vi "Analog Input - 1 Channel - N Samples.vi"() -> ()   [LabVIEW 2019]
uses:
  <vilib>/myRIO/Common/Instrument Driver Framework/ELVIS III v1.0/AI Block/vis/ELVIS III v1.0 AI Block Read.vi
  <vilib>/myRIO/Common/Instrument Driver Framework/ELVIS III v1.0/AI Block/vis/ELVIS III v1.0 Close AI Block.vi
  <vilib>/myRIO/Common/Instrument Driver Framework/myRIO v1.0/UART/vis/myRIO v1.0 Close UART.vi
  <vilib>/myRIO/Common/Instrument Driver Framework/Utilities/vis/Sample Rate To Ticks.vi
  <vilib>/myRIO/Common/Instrument Driver Framework/ELVIS III v1.0/AI Block/vis/ELVIS III v1.0 Unreserve AI Block.vi
  <vilib>/myRIO/Common/Instrument Driver Framework/ELVIS III v1.0/AI Block/vis/ELVIS III v1.0 Build MUX Configuration AI Block.vi
  <vilib>/Utility/error.llb/Error Cluster From Error Code.vi
  <vilib>/myRIO/Common/Instrument Driver Framework/myRIO v1.0/Resource Manager/vis/myRIO v1.0 Block Write Configuration.vi
  <vilib>/myRIO/Common/Instrument Driver Framework/ELVIS III v1.0/AI Block/vis/ELVIS III v1.0 AI Block Read Bank A.vi
  <vilib>/myRIO/Common/Instrument Driver Framework/ELVIS III v1.0/AI Block/vis/ELVIS III v1.0 AI Block Read Bank B.vi
  <vilib>/myRIO/Common/Instrument Driver Framework/ELVIS III v1.0/Resource Manager/vis/ELVIS III v1.0 Unreserve Channel List.vi
  <vilib>/myRIO/Common/Instrument Driver Framework/myRIO v1.0/myRIO v1.0 Close.vi
  <vilib>/myRIO/Common/Instrument Driver Framework/Utilities/vis/FPGA Ref Manager.vi
  <vilib>/myRIO/Common/Instrument Driver Framework/ELVIS III v1.0/ELVIS III v1.0 Reset FPGA.vi
  <vilib>/myRIO/Common/Instrument Driver Framework/myRIO v1.0/IRQ/vis/myRIO v1.0 IRQ Info FGV.vi
  <vilib>/myRIO/Common/Instrument Driver Framework/myRIO v1.0/IRQ/vis/myRIO v1.0 Timer IRQ Info FGV.vi
  <vilib>/myRIO/Common/Instrument Driver Framework/myRIO v1.0/IRQ/vis/myRIO v1.0 ISR Agent.vi
  <vilib>/myRIO/Instrument Drivers/Utilities/vis/Reset Index.vi
  <vilib>/myRIO/Common/Instrument Driver Framework/myRIO v1.0/Resource Manager/vis/myRIO v1.0 Block Write Resource Manager.vi
  <vilib>/myRIO/Instrument Drivers/Utilities/Utilities.lvlib
  <vilib>/myRIO/Instrument Drivers/Onboard IO/AI Block/AI Block.lvlib
panel:
  in  "Acquire Data":bool
  in  "Stop":bool
  out "Analog Data":dbl[](graph)
  # "ELVIS III Control IO"
  # "模拟输出单通道"
  # "Overview: Acquires N sample voltage values from Bank A, Channel 0 (A/AI0).\nInstructions:\n1. Connect A/AI0 to a valid signal.\n2. Run the VI.\n3. Click Acquire Data to trigger an acquisition."
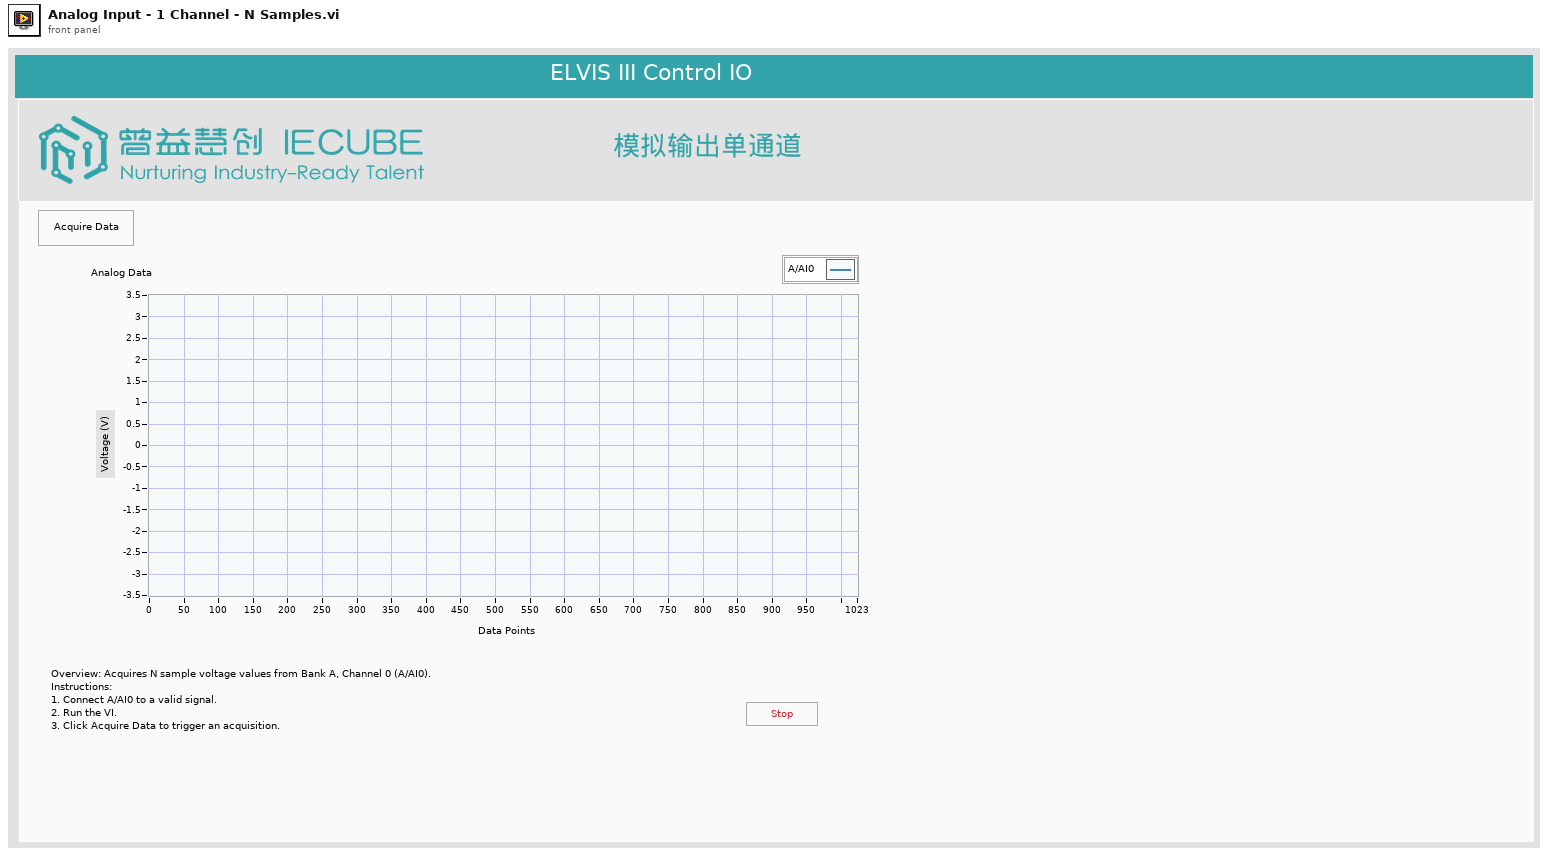
[diagram p1: front panel]
types:
  T1 = typedef "AI Block.lvlib/AI Block Reference.ctl" = cluster{"myRIO Reference":T2, "AI (N Samples) Channels List":T6, "AI (N Samples) Scaling Constants List":T8[]}
  T2 = typedef "myRIO Generic Hardware Reference.ctl" = cluster{"myRIO Model":T3, "myRIO Hardware Reference":T4}
  T3 = typedef "Hardware Version Enum.ctl" = enum16{"Unknown", "myRIO-1900", "myRIO-1950", "roboRIO", "NI ELVIS RIO CM", "ELVIS III"}
  T4 = typedef "myRIO v1.0 Reference.ctl" = cluster{"Generic FPGA Reference":T5, "Allow multiple opens":bool}
  T5 = typedef "Generic FPGA Reference.ctl" = refnum<k20>
  T6 = typedef "AI Block Channels List.ctl" = T7[]
  T7 = typedef "AI Block Channels Enum.ctl" = enum16{"Not Connected", "A/AI0 (N Samples)", "A/AI1 (N Samples)", "A/AI2 (N Samples)", "A/AI3 (N Samples)", "A/AI4 (N Samples)", "A/AI5 (N Samples)", "A/AI6 (N Samples)", "A/AI7 (N Samples)", "A/AI0 (DIFF N Samples)", "A/AI1 (DIFF N Samples)", "A/AI2 (DIFF N Samples)", "A/AI3 (DIFF N Samples)", "B/AI0 (N Samples)", "B/AI1 (N Samples)", "B/AI2 (N Samples)", "B/AI3 (N Samples)", "B/AI4 (N Samples)", "B/AI5 (N Samples)", "B/AI6 (N Samples)", "B/AI7 (N Samples)", "B/AI0 (DIFF N Samples)", "B/AI1 (DIFF N Samples)", "B/AI2 (DIFF N Samples)", "B/AI3 (DIFF N Samples)"}
  T8 = typedef "Analog Scaling Constants.ctl" = cluster{"LSB Weight (Volts)":dbl, "Offset (Volts)":dbl, "Signed?":bool}
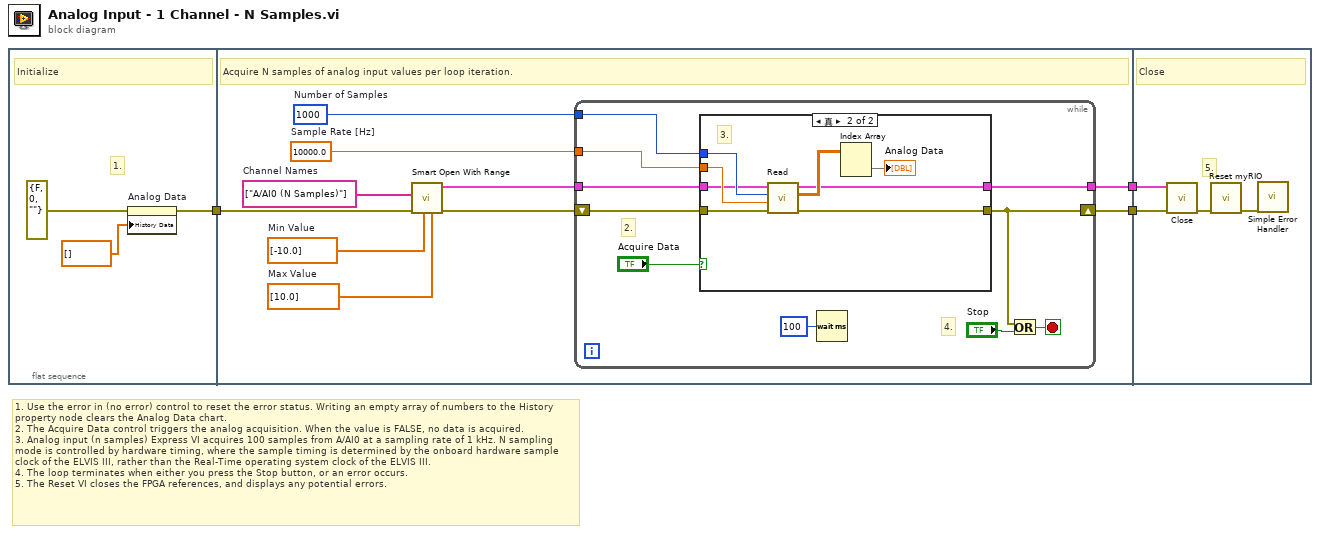
[diagram p0: block diagram]
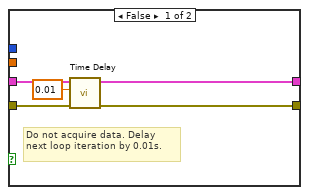
[diagram p2: hidden frame]
diagram:
  # "1. Use the error in (no error) control to reset the error status. Writing an empty array of numbers to the History property node clears the Analog Data chart. \n2. The Acquire Data control triggers the analog acquisition. When the value is FALSE, no data is acquired.\n3. Analog input (n samples) Express VI acquires 100 samples from A/AI0 at a sampling rate of 1 kHz. N sampling mode is controlled by hardware timing, where the sample timing is determined by the onboard hardware sample clock of the ELVIS III, rather than the Real-Time operating system clock of the ELVIS III. \n4. The loop terminates when either you press the Stop button, or an error occurs.\n5. The Reset VI closes the FPGA references, and displays any potential errors."
  n1 = flat-sequence {
    tunnel: [w6] -> w3
    tunnel: w3 -> [w8]
    tunnel: [w16] -> w2
    tunnel: [w9] -> w1
    tunnel: w2 -> [w40]
    tunnel: w1 -> [w41]
    frame #0 {
      # "1."
      # "Initialize"
      n2 = property on="Analog Data" class="WFChart (严格)"(error in=errorcluster {"status"=FALSE, "code"=0, "source"=""} ("Error In"), "History Data"=dbl[] []) -> (error out=w6:errorcluster)  [unwired: 1 in, 1 out]
    }
    frame #1 {
      w12 = 10000.0  # Sample Rate [Hz]
      w11 = u32 1000  # Number of Samples
      w15 = dbl[] [10.0]  # Max Value
      w14 = dbl[] [-10.0]  # Min Value
      w13 = tag[] ["A/AI0 (N Samples)"]  # Channel Names
      # "Acquire N samples of analog input values per loop iteration."
      n3 = call <vilib>:"Smart Open With Range.vi"("Max Value"=w15, "Min Value"=w14, "error in (no error)"=w8, "Channel Names"=w13) -> ("error out"=w7:errorcluster, "AI (N Samples) Ref Out"=w10:T1)  [unwired: 6 in]
      n4 = while {
        shift-right: [w23] -> w16
        shift-left: w7 -> [w17]
        tunnel: w12 -> [w22]
        tunnel: w11 -> [w21]
        tunnel: w10 -> [w20]
        tunnel: [w18] -> w9
        stop <- w24 stop-if-true
        # "4."
        # "2."
        n5 = case shown="真" "Acquire Data" {
          tunnel: [w30 w37] -> w23
          tunnel: w22 -> [_ w35]
          tunnel: w21 -> [_ w34]
          tunnel: w17 -> [w27 w33]
          tunnel: w20 -> [w28 w32]
          tunnel: [w28 w31] -> w18
          frame False {
            # "Do not acquire data. Delay next loop iteration by 0.01s."
            n6 = call "Time Delay"("error in (no error)"=w27, "Delay Time (s)"=0.01) -> ("error out"=w30:errorcluster)  [unwired: 9 in]
          }
          frame True {
            # "3."
            n7 = call <vilib>:"Read.vi"("error in (no error)"=w33, "Sample Rate [Hz]"=w35, "Number of Samples"=w34, "AI (N Samples) Ref In"=w32) -> ("error out"=w37:errorcluster, "Values"=w38:dbl[][], "AI (N Samples) Ref Out"=w31:T1)  [unwired: 5 in]
            n8 = Index Array(array=w38) -> (element=→"Analog Data":dbl[])  [unwired: 2 in]
          }
        }
        n9 = Wait (ms)(milliseconds to wait=u32 100 ("等待时间（毫秒）")) -> ()  [unwired: 1 out]
        n10 = Or(x=w23, y="Stop") -> (x .or. y?=w24:bool)
      }
    }
    frame #2 {
      # "5."
      # "Close"
      n11 = call <vilib>:"Close.vi"("error in (no error)"=w40, "AI (N Samples) Ref In"=w41) -> ("error out"=w39:errorcluster)  [unwired: 9 in]
      n12 = call <vilib>:"Reset myRIO.vi"("error in (no error)"=w39) -> ("error out"=w42:errorcluster)  [unwired: 10 in]
      n13 = call <vilib>:"Simple Error Handler.vi"("error in (no error)"=w42) -> ()  [unwired: 4 in, 5 out]
    }
  }
